vi "Bode Magnitude Plot.vi"() -> ()   [LabVIEW 2015]
uses:
  <vilib>/Analysis/NI_AALPro.lvlib
panel:
  out "XY Graph":cluster{"X":dbl, "Y":dbl}[](graph)
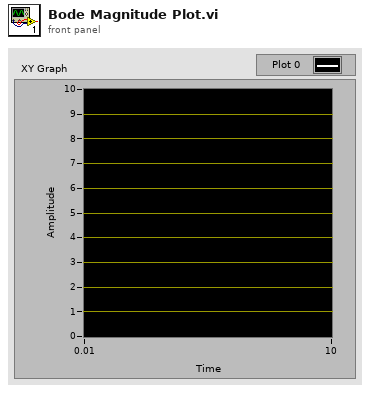
[diagram p1: front panel]
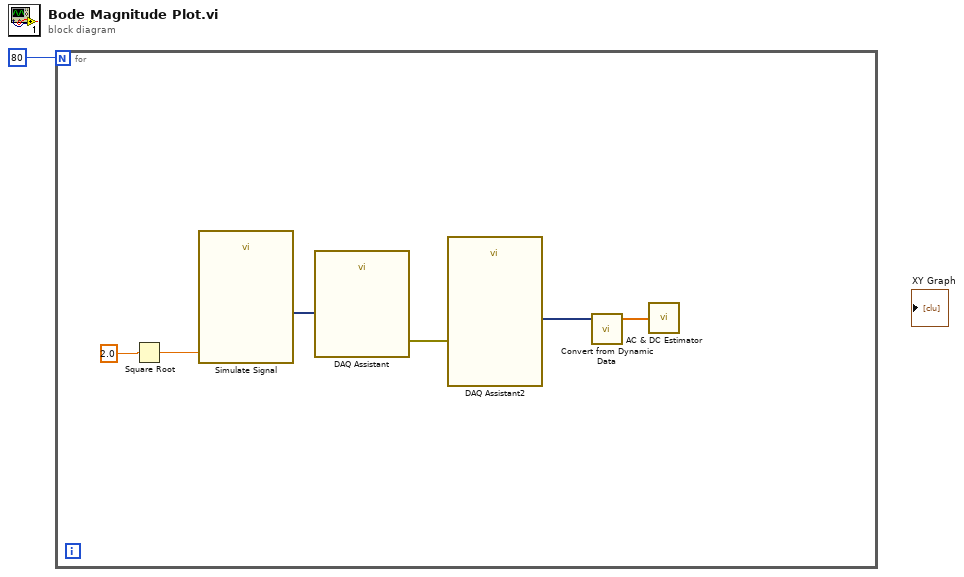
[diagram p0: block diagram]
diagram:
  n1 = for {
    N: 80 -> [_]
    n2 = Square Root(x=2.0) -> (sqrt(x)=w5:dbl)
    n3 = call "Simulate Signal"("Amplitude"=w5) -> ("Sine"=w7:dynamicdata)  [unwired: 13 in, 1 out]
    n4 = call "DAQ Assistant"("data"=w7) -> ("error out"=w6:errorcluster)  [unwired: 16 in, 2 out]
    n5 = call "DAQ Assistant2"("error in"=w6) -> ("data"=w3:dynamicdata)  [unwired: 16 in, 2 out]
    n6 = call "Convert from Dynamic Data"("Dynamic Data Type"=w3) -> ("Array"=w4:dbl[])  [unwired: 3 in]
    n7 = call <vilib>:"AC & DC Estimator.vi"("Signal (V)"=w4) -> ()  [unwired: 2 out]
  }
